vi "Pod Translation.vi"(8 "Y translation":dbl=1.0 format="%#_13g", 9 "X translation":dbl=1.0 format="%#_13g", 11 "Pod Coordinates":dbl[](array[numeric])) -> (3 "New Pod Coordinates":dbl[](array[numeric]))   [LabVIEW 2020]
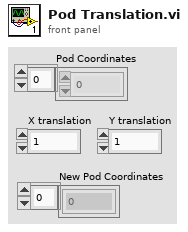
[diagram p1: front panel]
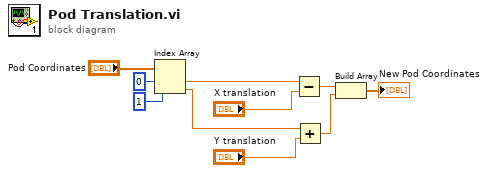
[diagram p0: block diagram]
diagram:
  n1 = Index Array(array="Pod Coordinates", index #1=0 ("index"), index #2=1 ("index")) -> (element #1=w5:dbl, element #2=w7:dbl)
  n2 = Subtract(x=w5, y="X translation") -> (x-y=w9:dbl)
  n3 = Add(x=w7, y="Y translation") -> (x+y=w10:dbl)
  n4 = Build Array(w9, w10) -> (→"New Pod Coordinates":dbl[])
